vi "RTS Build Listbox Data.vi"(8 "Error In":errorcluster, 10 "Full Data Set Input":string[][](array[string]), 11 "Point File in":T1[](array[typedef])) -> (0 "Error Out":errorcluster, 2 "Custom Titles":string[](array[string]), 3 "Custom Listbox Data":string[][](array[string]))   [LabVIEW 2016]
uses:
  Type Definitions/RTS Point File.ctl
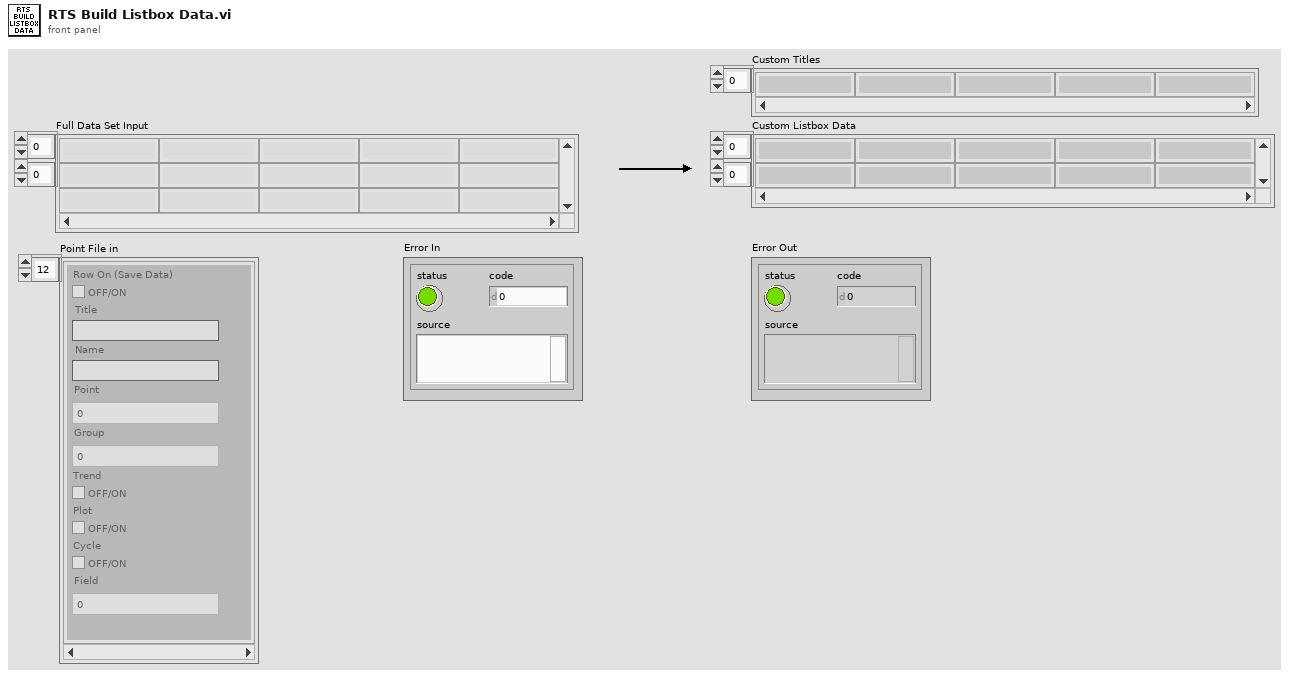
[diagram p1: front panel]
types:
  T1 = typedef "RTS Point File.ctl" = cluster{"Title":string, "Name":string, "Point":u8, "Plot":bool, "Trend":bool, "Cycle":bool, "Field":u8, "Row On (Save Data)":bool, "Group":u8}
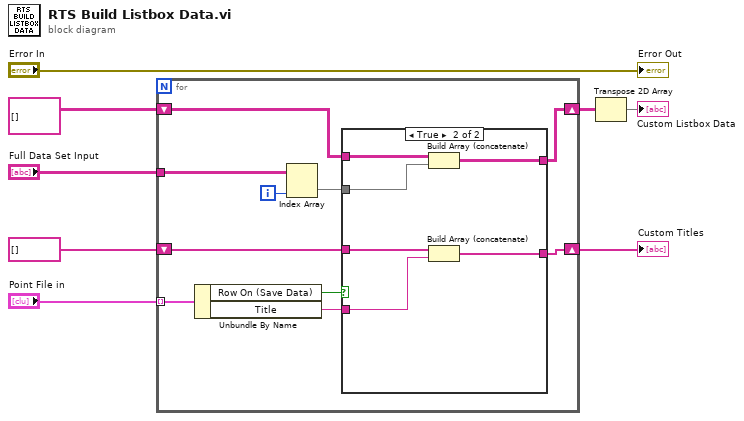
[diagram p0: block diagram]
diagram:
  n1 = for {
    tunnel: "Point File in" -> [w18] mode=indexing
    tunnel: "Full Data Set Input" -> [w16]
    shift-right: [w12] -> w6
    shift-left: string[][] [] -> [w13]
    shift-right: [w9] -> w1
    shift-left: string[] [] -> [w10]
    i -> [w15]
    n2 = Unbundle By Name(w18) -> ("Row On (Save Data)"=w17:bool, "Title"=w11:string)
    n3 = Index Array(array=w16, index (col)=w15) -> (element=w14:string[])  [unwired: 1 in]
    n4 = case shown="True" w17 {
      tunnel: w14 -> [_ w24]
      tunnel: w13 -> [w20 w26]
      tunnel: [w20 w25] -> w12
      tunnel: w11 -> [_ w21]
      tunnel: w10 -> [w19 w23]
      tunnel: [w19 w22] -> w9
      frame False {
      }
      frame True {
        n5 = Build Array (concatenate)(w26, w24) -> (w25:string[][])
        n6 = Build Array (concatenate)(w23, w21) -> (w22:string[])
      }
    }
  }
  "Custom Titles" <- w1
  n7 = Transpose 2D Array(2D array=w6) -> (transposed array=→"Custom Listbox Data":string[][])
  "Error Out" <- "Error In"
